vi "FTW-Logger-Process.vi"(0 "FTW Logger Configuration":T1="{\n  \"Identity\": \"EventLog\",\n  \"InboxAddress\": \"inproc://127.0.0.1:*\",\n  \"PublisherAddress\": \"\",\n  \"EnableInboxLogging\": false,\n  \"EnableJobLogging\": false,\n  \"ApplicationName\": \"Featherweight Application\",\n  \"LoggerDirectory\": \"[UserAppDir]//[ApplicationName]\",\n  \"LoggerDiskThrashDelay\": 200\n}", 11 "error in":errorcluster) -> (15 "error out":errorcluster)   [LabVIEW 2012, in "FTW-Actor.lvlib" / "FTW-Logger-Core.lvclass"]
uses:
  FTW-Logger-Core.lvclass
  Utility/FTW-Actor-Configuration.ctl
  FTW-Logger-Core.lvclass/FTW-Logger-Core.ctl
  Instance/FTW-ActorInstance.lvclass/FTW-ActorInstance.ctl
  JobSequencer/FTW-JobSequencer.lvclass/FTW-JobSequencer.ctl
  Core/Time/FTW-Time-DisplayFormat-Timestamp.ctl
  JobSequencer/FTW-SEQ-AddNext.vi
  FTW-Logger.lvclass
  Message/Request/FTW-Message-IncomingRequest.lvclass
  Instance/FTW-ActorInstance.lvclass
  FTW-Actor.lvlib
panel:
  # "Inputs"
  # "Outputs"
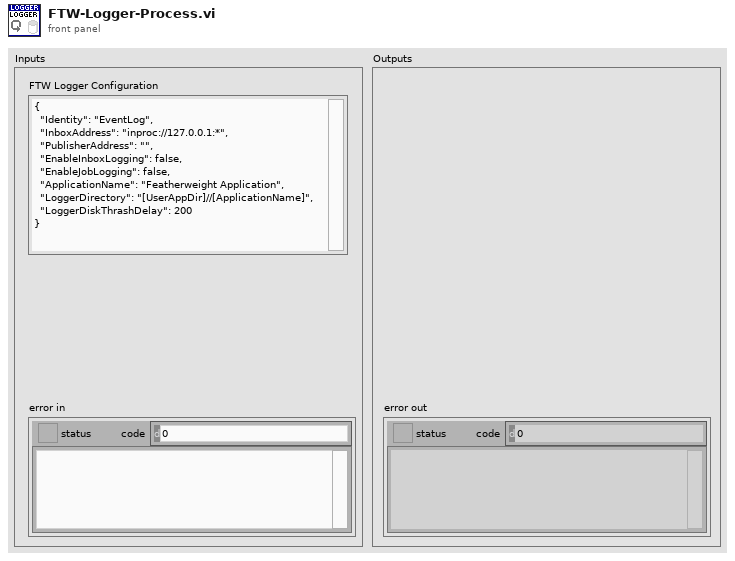
[diagram p1: front panel]
types:
  T1 = typedef "FTW-Actor.lvlib/FTW-Actor-Configuration.ctl" = string
  T2 = typedef "FTW-Time-DisplayFormat-Timestamp.ctl" = enum16{"YYYY-MM-DDT00:00:00.000Z (ISO-8601)", "YYYY-MM-DDT00-00-00Z (Simple ISO-8601)", "YYYY-MM-DD"}
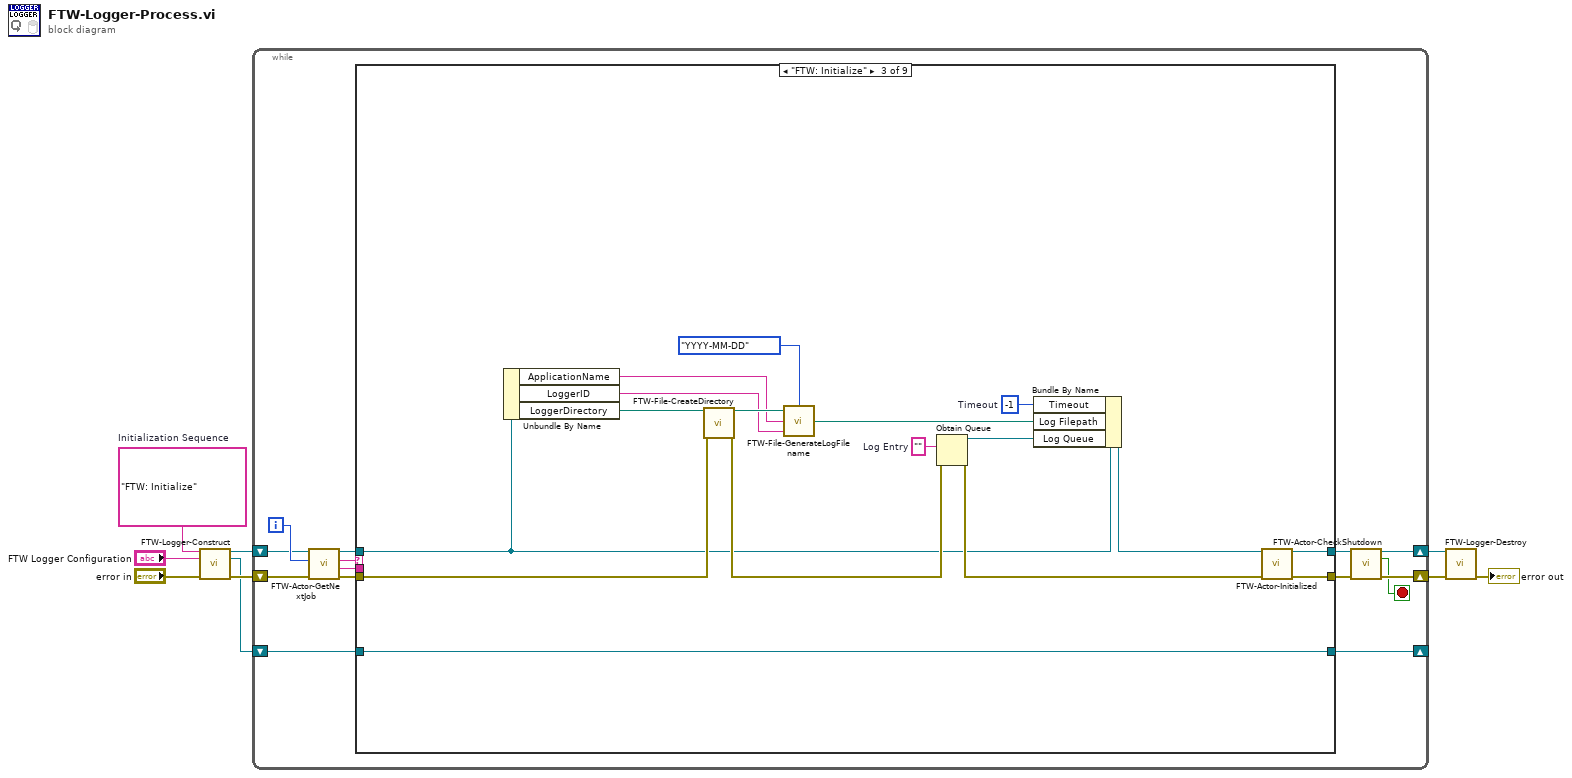
[diagram p0: block diagram]
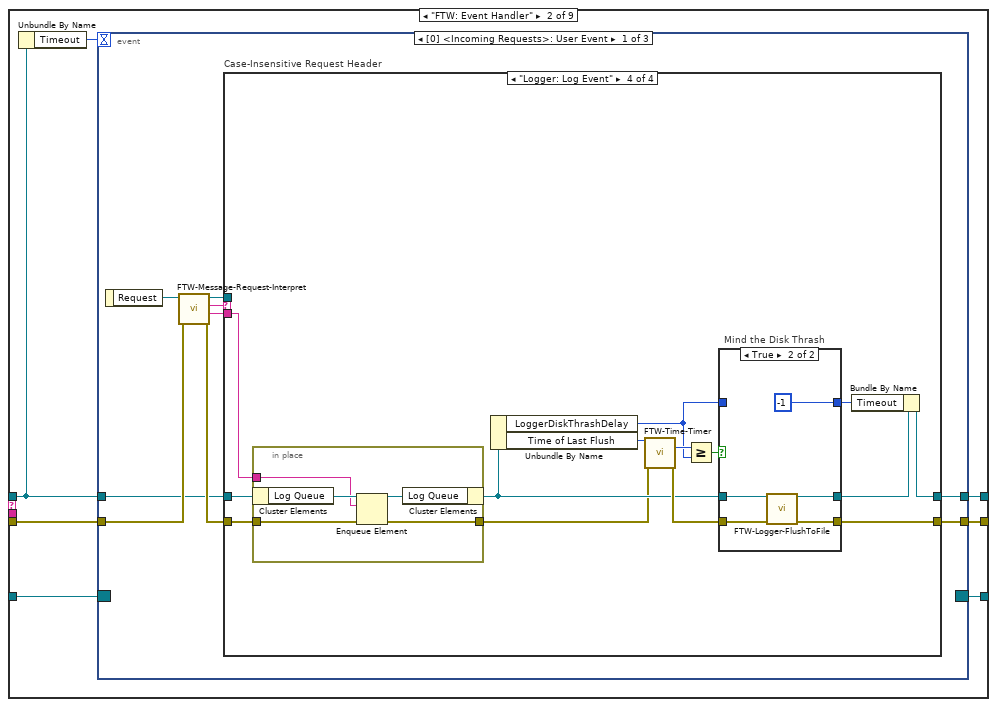
[diagram p3: hidden frame]
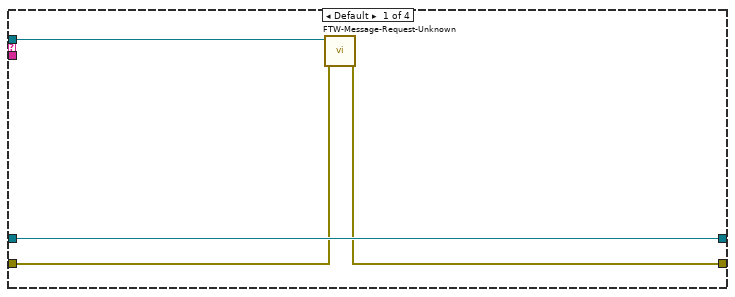
[diagram p4: hidden frame]
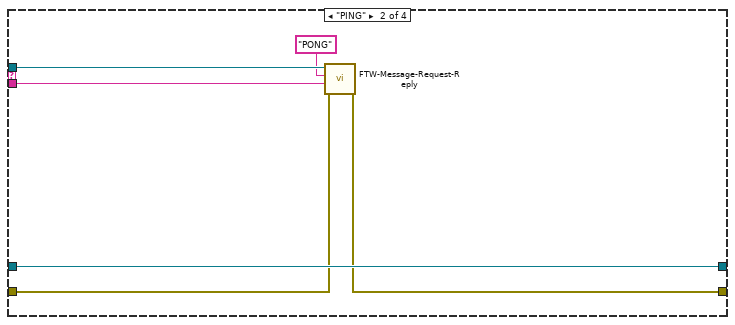
[diagram p5: hidden frame]
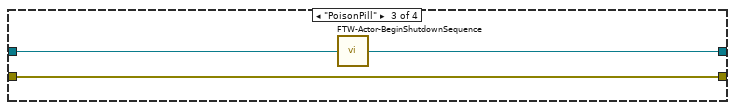
[diagram p6: hidden frame]
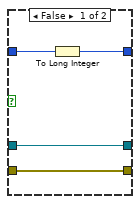
[diagram p7: hidden frame]
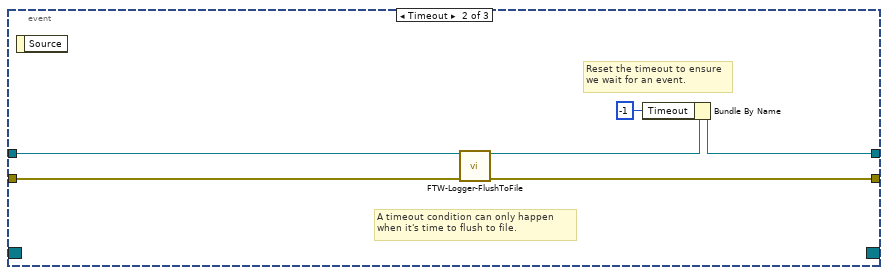
[diagram p8: hidden frame]
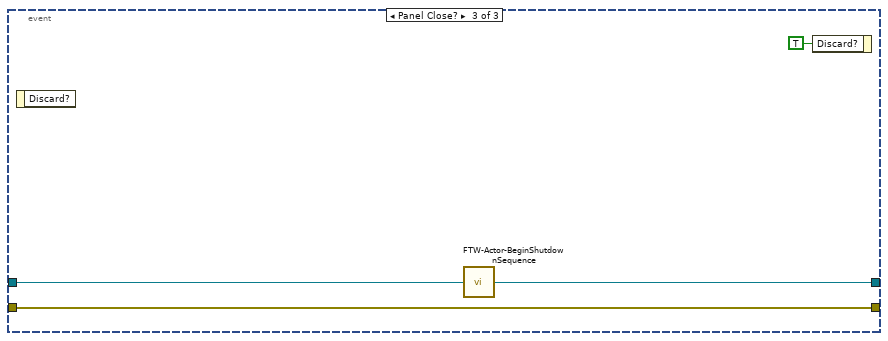
[diagram p9: hidden frame]
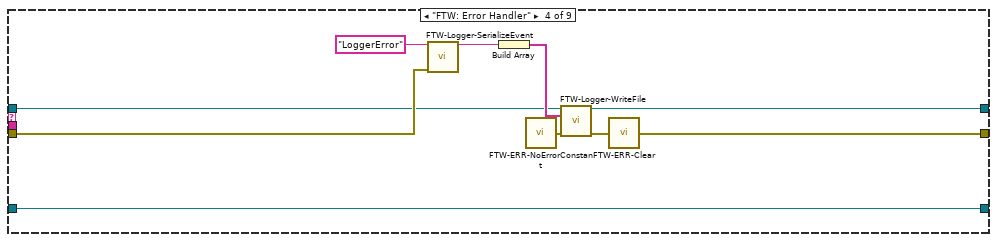
[diagram p10: hidden frame]
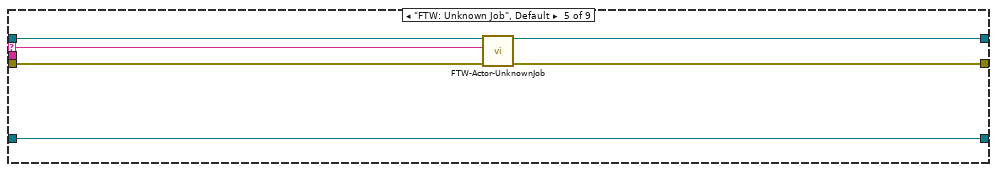
[diagram p11: hidden frame]
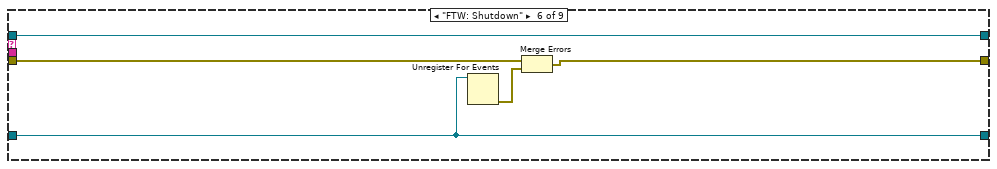
[diagram p12: hidden frame]
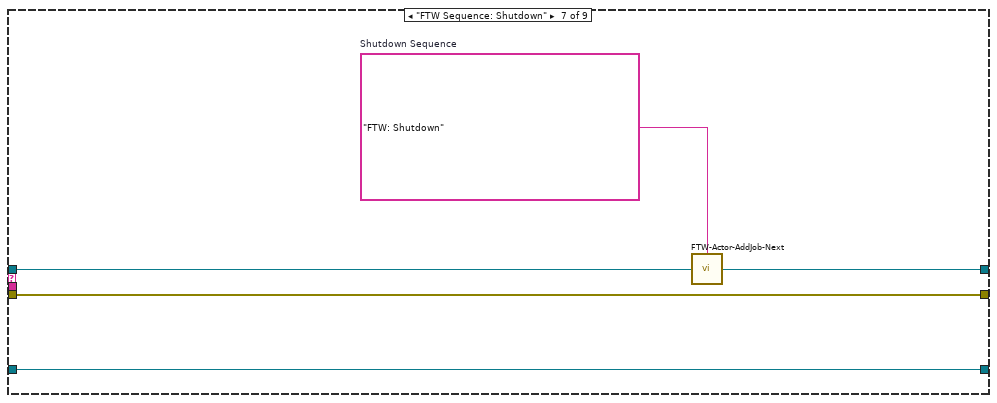
[diagram p13: hidden frame]
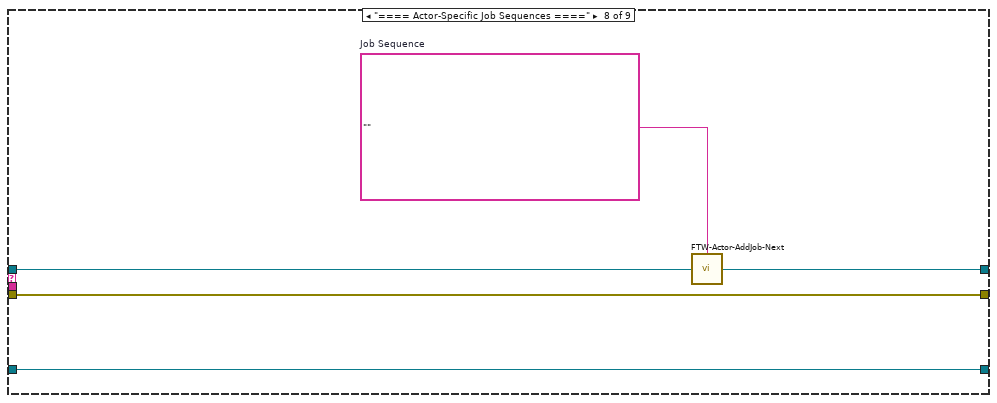
[diagram p14: hidden frame]
diagram:
  w2 = "FTW: Initialize"  # Initialization Sequence
  n1 = call "FTW-Logger-Construct.vi"("Initialization Sequence"=w2, "Logger Configuration"="FTW Logger Configuration", "error in"="error in") -> ("FTW Logger"=w6:refnum<class "FTW-Logger-Core.lvclass">, "Incoming Requests"=w3:refnum<event-registration>, "error out"=w5:errorcluster)  [unwired: 10 in]
  n2 = while {
    shift-right: [w12] -> w8
    shift-left: w5 -> [w21]
    shift-right: [w22] -> _
    shift-left: w3 -> [w23]
    shift-right: [w11] -> w9
    shift-left: w6 -> [w18]
    i -> [w20]
    stop <- w10 stop-if-true
    n3 = call "FTW-Actor-GetNextJob.vi"("error in"=w21, "Jobs Performed"=w20, "FTW Actor Instance"=w18) -> ("error out"=w19:errorcluster, "Job Data"=w15:string, "Job Name"=w16:string, "FTW Actor Instance out"=w17:refnum<class "FTW-Logger-Core.lvclass">)  [unwired: 5 in]
    n4 = case shown="\"FTW: Initialize\"" w16 {
      selector: w16 -> [_ _ _ _ w122 _ _ _ _]
      tunnel: [w25 w33 w102 w116 w123 w131 w135 w140 w144] -> w13
      tunnel: w19 -> [w25 w32 w107 w118 w121 w127 w135 w140 w144]
      tunnel: w23 -> [w26 w31 w105 w120 w126 w129 w136 w141 w143]
      tunnel: [w26 w30 w105 w120 w126 w129 w136 w141 w143] -> w22
      tunnel: w17 -> [w24 w27 w97 w112 w125 w128 w133 w138 w142]
      tunnel: [w24 w28 w103 w113 w124 w128 w132 w137 w142] -> w14
      tunnel: w15 -> [_ _ _ _ _ _ _ _ _]
      frame "==== Featherweight Framework Jobs ====" {
      }
      frame "FTW: Event Handler" {
        n5 = Unbundle By Name(w27) -> ("Timeout"=w29:i32)
        n6 = event shown="[0] <Incoming Requests>: User Event" {
          selector: w31 -> [_ _ _]
          dyn-events: [_ _ _] -> w30
          timeout: w29 -> [_ _ _]
          tunnel: [w40 w88 w92] -> w33
          tunnel: w32 -> [w41 w89 w92]
          tunnel: [w39 w84 w90] -> w28
          tunnel: w27 -> [w38 w87 w91]
          event User Event {
            n7 = event-data() -> ("Request"=w35:refnum<class "FTW-Message-IncomingRequest.lvclass">)  [unwired: 1 in]
            n8 = call "FTW-Message-Request-Interpret.vi"("error in"=w41, "FTW Incoming Request"=w35) -> ("error out"=w42:errorcluster, "Request Body"=w36:string, "Request Header"=w37:string, "FTW Request"=w34:refnum<class "FTW-Message-IncomingRequest.lvclass">)  [unwired: 6 in]
            n9 = case "Case-Insensitive Request Header" shown="\"Logger: Log Event\"" w37 {
              tunnel: [w43 w50 w55 w66] -> w40
              tunnel: w42 -> [w44 w51 w55 w59]
              tunnel: [w46 w52 w53 w62] -> w39
              tunnel: w38 -> [w46 w52 w54 w61]
              tunnel: w36 -> [_ w47 _ w57]
              tunnel: w34 -> [w45 w49 _ _]
              frame Default {
                n10 = call "FTW-Message-Request-Unknown.vi"("error in"=w44, "FTW Incoming Request"=w45) -> ("error out"=w43:errorcluster)  [unwired: 9 in]
              }
              frame "PING" {
                n11 = call "FTW-Message-Request-Reply.vi"("error in"=w51, "Response Body"=w47, "Response Header"="PONG", "FTW Incoming Request"=w49) -> ("error out"=w50:errorcluster)  [unwired: 6 in, 1 out]
              }
              frame "PoisonPill" {
                n12 = call "FTW-Actor-BeginShutdownSequence.vi"("FTW Actor Instance"=w54) -> ("FTW Actor Instance out"=w53:refnum<class "FTW-Logger-Core.lvclass">)  [unwired: 3 in]
              }
              frame "Logger: Log Event" {
                n13 = in-place {
                  in-place-border: w59 -> [w74]
                  in-place-border: [w71] -> w58
                  in-place-border: w57 -> [w70]
                  n14 = in-place-cluster #1(w61) -> ("Log Queue"=w73:refnum<queue>)
                  n15 = Enqueue Element(queue=w73, element=w70, error in (no error)=w74) -> (queue out=w72:refnum<queue>, error out=w71:errorcluster)  [unwired: 1 in, 1 out]
                  n16 = in-place-cluster #1("Log Queue"=w72) -> (w60:refnum<class "FTW-Logger-Core.lvclass">)
                }
                n17 = Unbundle By Name(w60) -> ("LoggerDiskThrashDelay"=w56:u32, "Time of Last Flush"=w69:u32)
                n18 = call "FTW-Time-Timer.vi"("Initial Tick Count"=w69, "error in"=w58) -> ("Elapsed Time"=w68:u32, "error out"=w67:errorcluster)  [unwired: 11 in, 1 out]
                n19 = Greater Or Equal?(x=w68, y=w56) -> (x >= y?=w65:bool)
                n20 = case "Mind the Disk Thrash" shown="True" w65 {
                  tunnel: [w78 w80] -> w63
                  tunnel: w60 -> [w78 w81]
                  tunnel: w67 -> [w77 w83]
                  tunnel: [w77 w82] -> w66
                  tunnel: [w75 -1 ("Timeout")] -> w64
                  tunnel: w56 -> [w76 _]
                  frame False {
                    n21 = To Long Integer(number=w76) -> (32bit integer=w75:i32)
                  }
                  frame True {
                    n22 = call "FTW-Logger-FlushToFile.vi"("FTW Logger"=w81, "error in"=w83) -> ("FTW Logger out"=w80:refnum<class "FTW-Logger-Core.lvclass">, "error out"=w82:errorcluster)  [unwired: 12 in]
                  }
                }
                n23 = Bundle By Name(cluster=w63, "Timeout"=w64) -> (w62:refnum<class "FTW-Logger-Core.lvclass">)
              }
            }
          }
          event Timeout {
            # "Reset the timeout to ensure\nwe wait for an event."
            # "A timeout condition can only happen\nwhen it's time to flush to file."
            n24 = event-data() -> ()  [unwired: 1 in, 1 out]
            n25 = call "FTW-Logger-FlushToFile.vi"("FTW Logger"=w87, "error in"=w89) -> ("FTW Logger out"=w85:refnum<class "FTW-Logger-Core.lvclass">, "error out"=w88:errorcluster)  [unwired: 12 in]
            n26 = Bundle By Name(cluster=w85, "Timeout"=-1) -> (w84:refnum<class "FTW-Logger-Core.lvclass">)
          }
          event Panel Close? {
            n27 = event-data() -> ()  [unwired: 1 in, 1 out]
            n28 = call "FTW-Actor-BeginShutdownSequence.vi"("FTW Actor Instance"=w91) -> ("FTW Actor Instance out"=w90:refnum<class "FTW-Logger-Core.lvclass">)  [unwired: 3 in]
            n29 = event-data("Discard?"=TRUE) -> ()  [unwired: 1 in, 1 out]
          }
        }
      }
      frame "FTW: Initialize" {
        w98 = ""  # Log Entry
        w108 = -1  # Timeout
        n30 = Unbundle By Name(w97) -> ("ApplicationName"=w96:string, "LoggerID"=w95:string, "LoggerDirectory"=w94:path)
        n31 = call "FTW-File-CreateDirectory.vi"("Directory to Create"=w94, "error in"=w107) -> ("Created Directory"=w106:path, "error out"=w100:errorcluster)  [unwired: 12 in]
        n32 = call "FTW-File-GenerateLogFilename.vi"("Date Format"=FTW-Time-DisplayFormat-Timestamp."YYYY-MM-DD", "Type"=w95, "Application"=w96, "Directory"=w106) -> ("Filepath"=w110:path)
        n33 = Obtain Queue(element data type=w98, error in (no error)=w100) -> (queue out=w101:refnum<queue>, error out=w99:errorcluster)  [unwired: 3 in, 1 out]
        n34 = Bundle By Name(cluster=w97, "Timeout"=w108, "Log Filepath"=w110, "Log Queue"=w101) -> (w104:refnum<class "FTW-Logger-Core.lvclass">)
        n35 = call-dynamic "FTW-Actor-Initialized.vi"("FTW Actor Instance"=w104, "error in"=w99) -> ("FTW Actor Instance out"=w103:refnum<class "FTW-Logger-Core.lvclass">, "error out"=w102:errorcluster)  [unwired: 12 in]
      }
      frame "FTW: Error Handler" {
        n36 = call "FTW-Logger-SerializeEvent.vi"("Event Type"="LoggerError", "Error to Log"=w118) -> ("Serialized Event"=w115:string)  [unwired: 13 in]
        n37 = Build Array(w115) -> (w114:string[])
        n38 = call "FTW-ERR-NoErrorConstant.vi"() -> ("no error"=w111:errorcluster)
        n39 = call "FTW-Logger-WriteFile.vi"("FTW Logger"=w112, "Entries to Log"=w114, "error in"=w111) -> ("FTW Logger out"=w113:refnum<class "FTW-Logger-Core.lvclass">, "error out"=w117:errorcluster)  [unwired: 11 in]
        n40 = call "FTW-ERR-Clear.vi"("error to snuff"=w117) -> ("no error"=w116:errorcluster)
      }
      frame "FTW: Unknown Job", Default {
        n41 = call-dynamic "FTW-Actor-UnknownJob.vi"("FTW Actor Instance"=w125, "Unknown Job"=w122, "error in"=w121) -> ("FTW Actor Instance out"=w124:refnum<class "FTW-Logger-Core.lvclass">, "error out"=w123:errorcluster)  [unwired: 11 in]
      }
      frame "FTW: Shutdown" {
        n42 = Unregister For Events(event registration refnum=w129) -> (error out=w130:errorcluster)  [unwired: 1 in]
        n43 = Merge Errors(w127, w130) -> (w131:errorcluster)
      }
      frame "FTW Sequence: Shutdown" {
        w134 = "FTW: Shutdown"  # Shutdown Sequence
        n44 = call "FTW-Actor-AddJob-Next.vi"("Add Next in Job Queue"=w134, "FTW Actor Instance"=w133) -> ("FTW Actor Instance out"=w132:refnum<class "FTW-Logger-Core.lvclass">)  [unwired: 2 in]
      }
      frame "==== Actor-Specific Job Sequences ====" {
        w139 = ""  # Job Sequence
        n45 = call "FTW-Actor-AddJob-Next.vi"("Add Next in Job Queue"=w139, "FTW Actor Instance"=w138) -> ("FTW Actor Instance out"=w137:refnum<class "FTW-Logger-Core.lvclass">)  [unwired: 2 in]
      }
      frame "==== Actor-Specific Jobs ====" {
      }
    }
    n46 = call "FTW-Actor-CheckShutdown.vi"("FTW Actor Instance"=w14, "error in"=w13) -> ("FTW Actor Instance out"=w11:refnum<class "FTW-Logger-Core.lvclass">, "Shutdown?"=w10:bool, "error out"=w12:errorcluster)  [unwired: 11 in]
  }
  n47 = call "FTW-Logger-Destroy.vi"("FTW Logger"=w9, "error in"=w8) -> ("error out"=→"error out":errorcluster)  [unwired: 13 in]
